vi "GetImage.vi"(0 "XRef":T13, 1 "State In":T3) -> (14 "Image":T2, 15 "Fatal Error Out":T1)   [LabVIEW 2020, in "Parallel Diagram Block.xnode"]
uses:
  Parallel Diagram Block.xnode
  <vilib>/XNodeSupport/XNodeXNodeRef.ctl
  <vilib>/XNodeSupport/NI_XNodeSupport.lvlib
  <vilib>/XNodeSupport/XNodeImage.ctl
  <vilib>/XNodeSupport/XNodeErrorCluster.ctl
  State.ctl
  Parallel Block/Value Type.ctl
  Parallel Block/Parallel Block.lvlib
  Parallel Block/Type Descriptor.ctl
  <vilib>/picture/picture.llb/imagedata.ctl
  Parallel Block/Direction.ctl
  Parallel Block/Terminal Mode.ctl
  Parallel Block/Terminal Type.ctl
  Parallel Block/Type Mode.ctl
  Parallel Block/Value Mode.ctl
  Parallel Block/Manager Node.ctl
panel:
  out "Picture":picture
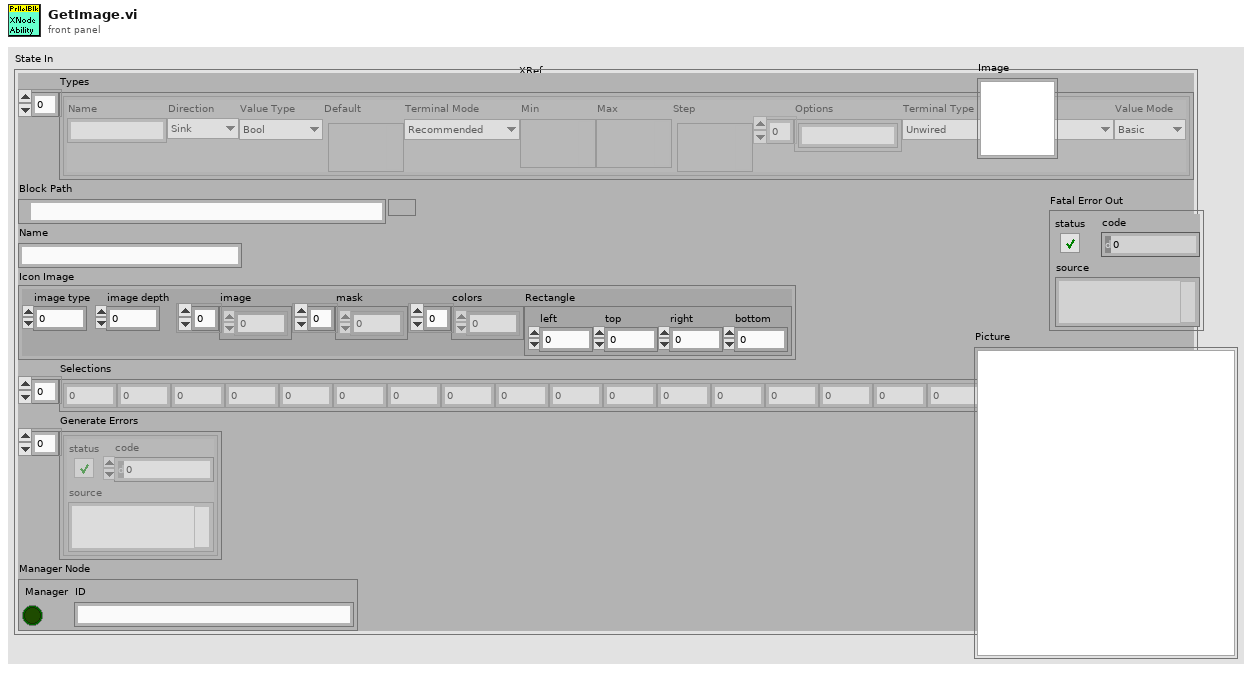
[diagram p1: front panel]
types:
  T1 = typedef "NI_XNodeSupport.lvlib/XNodeErrorCluster.ctl" = errorcluster
  T2 = typedef "NI_XNodeSupport.lvlib/XNodeImage.ctl" = picture
  T3 = typedef "Parallel Diagram Block.xnode/State.ctl" = cluster{"Types":T4[], "Block Path":path, "Name":string, "Icon Image":T11, "Selections":i32[], "Generate Errors":errorcluster[], "Manager Node":T12}
  T4 = typedef "Parallel Block.lvlib/Type Descriptor.ctl" = cluster{"Name":string, "Direction":T5, "Value Type":T6, "Default":variant, "Terminal Mode":T7, "Min":variant, "Max":variant, "Step":variant, "Options":string[], "Terminal Type":T8, "Type Mode":T9, "Value Mode":T10}
  T5 = typedef "Parallel Block.lvlib/Direction.ctl" = enum16{"Sink", "Source"}
  T6 = typedef "Parallel Block.lvlib/Value Type.ctl" = enum16{"Unknown", "Bool", "U8", "U16", "U32", "U64", "I8", "I16", "I32", "I64", "SGL", "DBL", "CSG", "CDB", "CDBWfm", "String", "DBLWfm"}
  T7 = typedef "Parallel Block.lvlib/Terminal Mode.ctl" = enum16{"Recommended", "Required", "None"}
  T8 = typedef "Parallel Block.lvlib/Terminal Type.ctl" = enum16{"Unwired", "BadType", "Connection", "Value", "Control Ref", "BadRefType"}
  T9 = typedef "Parallel Block.lvlib/Type Mode.ctl" = enum16{"Output", "Single - Strict", "Single - Coerced", "Stream"}
  T10 = typedef "Parallel Block.lvlib/Value Mode.ctl" = enum16{"Basic", "Range", "Select"}
  T11 = typedef "imagedata.ctl" = cluster{"image type":i32, "image depth":i32, "image":u8[], "mask":u8[], "colors":u32[], "Rectangle":cluster{"left":i16, "top":i16, "right":i16, "bottom":i16}}
  T12 = typedef "Parallel Block.lvlib/Manager Node.ctl" = cluster{"Manager":bool, "ID":string}
  T13 = typedef "NI_XNodeSupport.lvlib/XNodeXNodeRef.ctl" = refnum<vi>
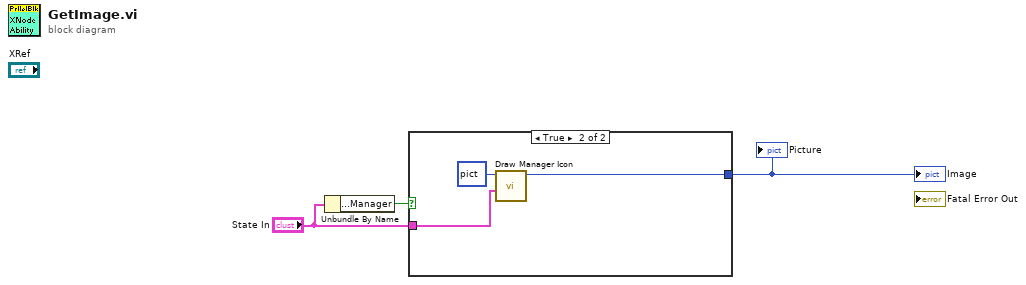
[diagram p0: block diagram]
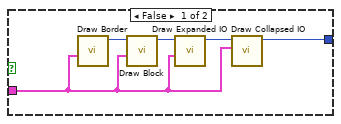
[diagram p2: hidden frame]
diagram:
  n1 = Unbundle By Name("State In") -> ("Manager Node.Manager"=w1:bool)
  n2 = case shown="True" w1 {
    tunnel: [w5 w11] -> w3
    tunnel: "State In" -> [w4 w10]
    frame False {
      n3 = call "Draw Border.vi"("State"=w4) -> ("Picture"=w8:picture)  [unwired: 10 in]
      n4 = call "Draw Block.vi"("State"=w4, "Picture In"=w8) -> ("Picture"=w7:picture)  [unwired: 9 in]
      n5 = call "Draw Expanded IO.vi"("State"=w4, "Picture In"=w7) -> ("Picture"=w6:picture)  [unwired: 9 in]
      n6 = call "Draw Collapsed IO.vi"("State"=w4, "Picture In"=w6) -> ("Picture"=w5:picture)  [unwired: 9 in]
    }
    frame True {
      n7 = call "Draw Manager Icon.vi"("State"=w10, "Picture In"=picture data[5B]) -> ("Picture"=w11:picture)  [unwired: 9 in]
    }
  }
  "Image" <- w3
  "Picture" <- w3
